vi "Bottom Visible.vi"(8 "Current column":i32, 9 "Current row":i32, 10 "Full array":i32[][](array[numeric]), 11 "Element":i32) -> (2 "Viewing Distance":i32, 3 "Visible":bool)   [LabVIEW 2021]
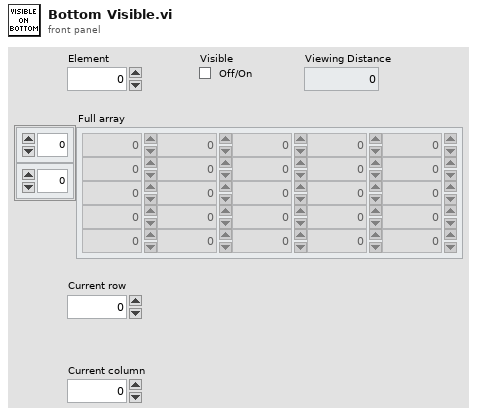
[diagram p1: front panel]
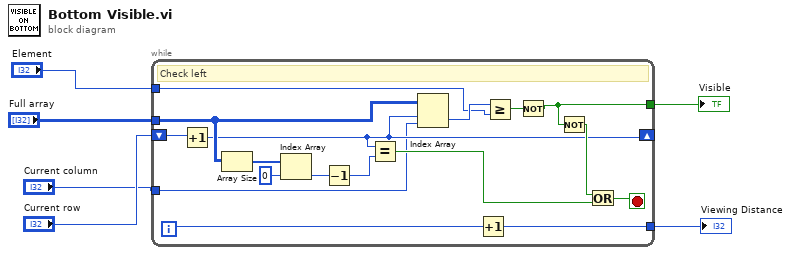
[diagram p0: block diagram]
diagram:
  n1 = while {
    shift-right: [w10] -> _
    shift-left: "Current row" -> [w20]
    tunnel: "Element" -> [w12]
    tunnel: "Full array" -> [w19]
    tunnel: "Current column" -> [w9]
    tunnel: [w11] -> w6
    tunnel: [w7] -> w1
    i -> [w8]
    stop <- w21 stop-if-true
    # "Check left"
    n2 = Increment(x=w20) -> (x+1=w10:i32)
    n3 = Array Size(array=w19) -> (size(s)=w18:i32[])
    n4 = Index Array(array=w18, index=0) -> (element=w17:i32)
    n5 = Decrement(x=w17) -> (x-1=w16:i32)
    n6 = Equal?(x=w10, y=w16) -> (x = y?=w22:bool)
    n7 = Index Array(array=w19, index (row)=w10, index (col)=w9) -> (element=w13:i32)
    n8 = Increment(x=w8) -> (x+1=w7:i32)
    n9 = Greater Or Equal?(x=w13, y=w12) -> (x >= y?=w14:bool)
    n10 = Not(x=w14) -> (.not. x?=w11:bool)
    n11 = Not(x=w11) -> (.not. x?=w23:bool)
    n12 = Or(x=w23, y=w22) -> (x .or. y?=w21:bool)
  }
  "Visible" <- w6
  "Viewing Distance" <- w1
